vi "Historical Data Access Server.vi"() -> ()   [LabVIEW 2019, in "OPC UA Demo.lvlib"]
doc: "Demonstrates the use of the <B>OPC UA Historical Data Access</B> functionality as an OPC UA server."
uses:
  OPC UA Demo.lvlib
  <vilib>/OPCUA/controls/Data Type.ctl
  <vilib>/OPCUA/controls/Historical Access.ctl
  <vilib>/OPCUA/server/Write Double.vi
  <vilib>/OPCUA/NI OPC UA Server.lvlib
  <vilib>/ptbypt/NI_PtbyPt.lvlib
panel:
  out "Node0":dbl(graph)
  out "Node1":dbl(graph)
  in  "queue size":u32=2000
  in  "stop":bool
  out "Node2":dbl(graph)
  out "server endpoint URL":string
  # "Overview: Demonstrates the use of the OPC UA Historical Data Access functionality as an OPC UA server.\nRequirements: \n1. LabVIEW OPC UA Toolkit\n2. Run this VI on RT targets or Windows\nInstructions:\n1. Adjust queue size to change the buffer size of history data.\n2. Run the VI.\n3. Run Historical Data Access Client.vi in OPC UA Demo.lvproj."
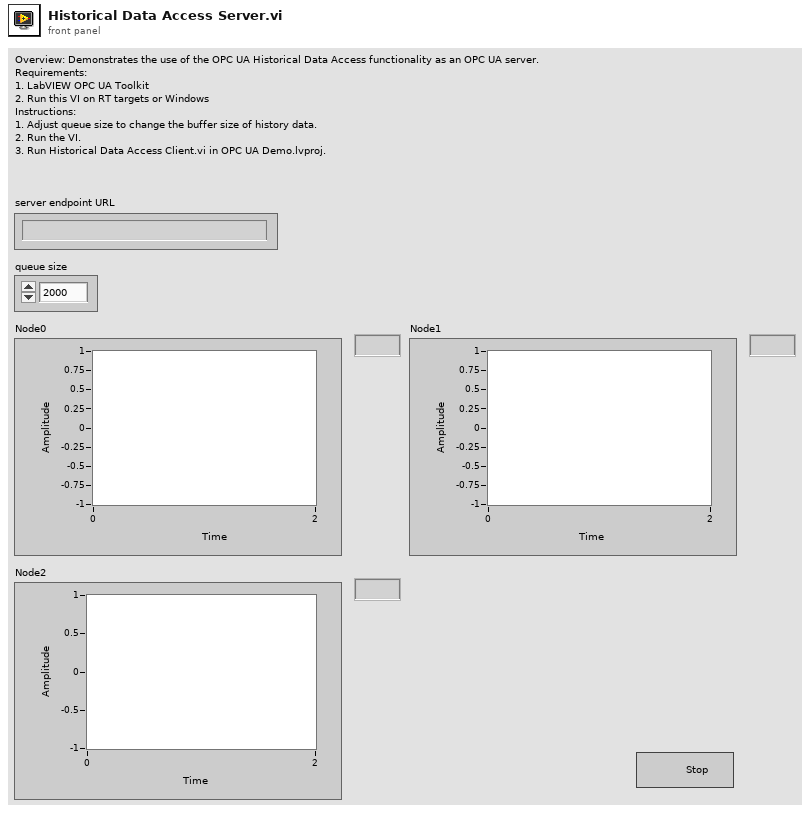
[diagram p1: front panel]
types:
  T1 = typedef "Historical Access.ctl" = cluster{"enable":bool, "queue size (1000)":u32}
  T2 = typedef "Data Type.ctl" = u16
  T3 = cluster{"name":string, "data type":T2, "access level":u16, "description":string}
  T4 = typedef "OPC UA Server Refnum.ctl" = refnum<k21>
  T5 = typedef "NodeId.ctl" = string
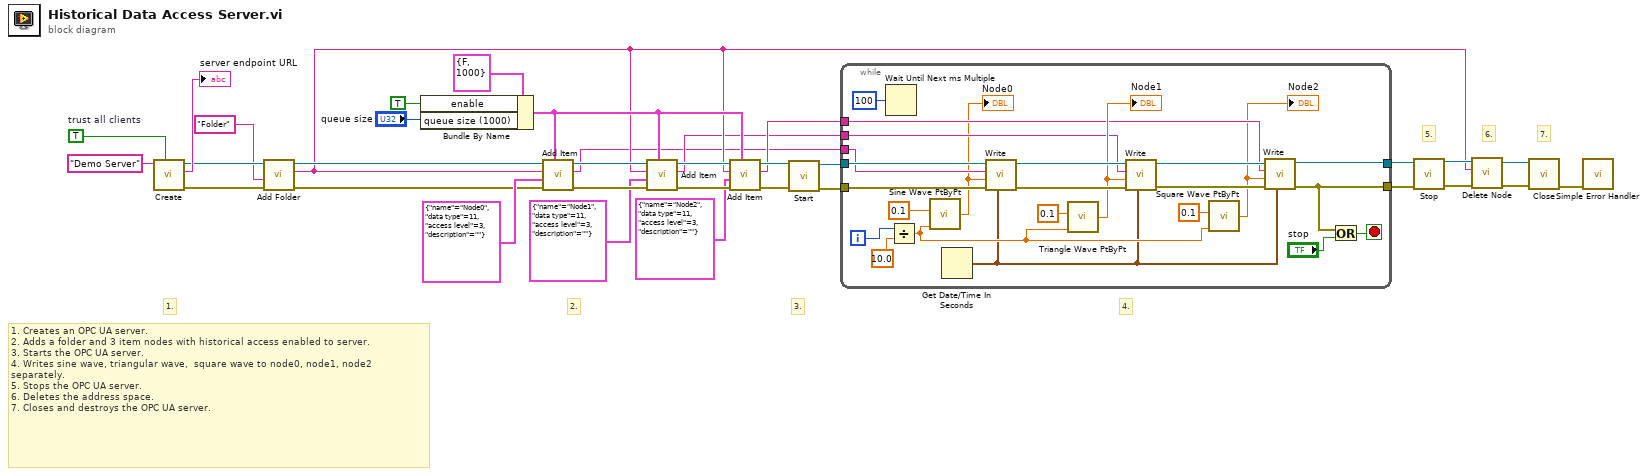
[diagram p0: block diagram]
diagram:
  w1 = TRUE  # trust all clients
  # "7."
  # "6."
  # "5."
  # "4."
  # "3."
  # "2."
  # "1."
  # "1. Creates an OPC UA server.\n2. Adds a folder and 3 item nodes with historical access enabled to server.\n3. Starts the OPC UA server.\n4. Writes sine wave, triangular wave,  square wave to node0, node1, node2 separately. \n5. Stops the OPC UA server.\n6. Deletes the address space.\n7. Closes and destroys the OPC UA server."
  n1 = call <vilib>:"Create.vi"("trust all clients (F)"=w1, "OPC UA server name"="Demo Server") -> ("error out"=w31:errorcluster, "server endpoint URL"=→"server endpoint URL":string, "OPC UA server refnum out"=w32:T4)  [unwired: 7 in]
  n2 = call <vilib>:"Add Folder.vi"("error in (no error)"=w31, "folder name"="Folder", "OPC UA server refnum in"=w32) -> ("error out"=w27:errorcluster, "folder node ID"=w6:T5, "OPC UA server refnum out"=w28:T4)  [unwired: 5 in]
  n3 = Bundle By Name(cluster=T1 {"enable"=FALSE, "queue size (1000)"=1000} ("historical access"), "enable"=TRUE, "queue size (1000)"="queue size") -> (w11:T1)
  n4 = call <vilib>:"Add Item.vi"("historical access"=w11, "error in (no error)"=w27, "item"=T3 {"name"="Node0", "data type"=11, "access level"=3, "description"=""}, "parent folder node ID"=w6, "OPC UA server refnum in"=w28) -> ("error out"=w15:errorcluster, "item node ID"=w2:T5, "OPC UA server refnum out"=w14:T4)  [unwired: 2 in, 1 out]
  n5 = call <vilib>:"Add Item.vi"("historical access"=w11, "error in (no error)"=w15, "item"=T3 {"name"="Node1", "data type"=11, "access level"=3, "description"=""}, "parent folder node ID"=w6, "OPC UA server refnum in"=w14) -> ("error out"=w8:errorcluster, "item node ID"=w3:T5, "OPC UA server refnum out"=w12:T4)  [unwired: 2 in, 1 out]
  n6 = call <vilib>:"Add Item.vi"("historical access"=w11, "error in (no error)"=w8, "item"=T3 {"name"="Node2", "data type"=11, "access level"=3, "description"=""}, "parent folder node ID"=w6, "OPC UA server refnum in"=w12) -> ("error out"=w9:errorcluster, "item node ID"=w4:T5, "OPC UA server refnum out"=w10:T4)  [unwired: 2 in, 1 out]
  n7 = call <vilib>:"Start.vi"("error in (no error)"=w9, "OPC UA server refnum in"=w10) -> ("error out"=w23:errorcluster, "OPC UA server refnum out"=w24:T4)  [unwired: 7 in, 1 out]
  n8 = while {
    tunnel: w24 -> [w58]
    tunnel: w23 -> [w56]
    tunnel: [w38] -> w25
    tunnel: [w48] -> w26
    tunnel: w4 -> [w41]
    tunnel: w3 -> [w42]
    tunnel: w2 -> [w43]
    i -> [w55]
    stop <- w39 stop-if-true
    n9 = Wait Until Next ms Multiple(millisecond multiple=u32 100) -> ()  [unwired: 1 out]
    n10 = Divide(x=w55, y=10.0 ("frequency")) -> (x/y=w46:dbl)
    n11 = call <vilib>:"Sine Wave PtByPt.vi"("time"=w46, "frequency"=0.1) -> ("sine wave"=w36:dbl)  [unwired: 2 in]
    "Node0" <- w36
    n12 = Get Date/Time In Seconds() -> (seconds since 1Jan1904=w37:timestamp)
    n13 = call-poly <vilib>:"Write.vi"("timestamp (current time)"=w37, "error in (no error)"=w56, "value"=w36, "node ID"=w43, "OPC UA server refnum in"=w58) -> ("error out"=w51:errorcluster, "OPC UA server refnum out"=w52:T4)  [unwired: 4 in, 1 out]
    n14 = call <vilib>:"Triangle Wave PtByPt.vi"("time"=w46, "frequency"=0.1) -> ("triangle wave"=w44:dbl)  [unwired: 2 in]
    "Node1" <- w44
    n15 = call-poly <vilib>:"Write.vi"("timestamp (current time)"=w37, "error in (no error)"=w51, "value"=w44, "node ID"=w42, "OPC UA server refnum in"=w52) -> ("error out"=w50:errorcluster, "OPC UA server refnum out"=w49:T4)  [unwired: 4 in, 1 out]
    n16 = call <vilib>:"Square Wave PtByPt.vi"("frequency"=0.1, "time"=w46) -> ("square wave"=w35:dbl)  [unwired: 3 in]
    "Node2" <- w35
    n17 = call-poly <vilib>:"Write.vi"("timestamp (current time)"=w37, "error in (no error)"=w50, "value"=w35, "node ID"=w41, "OPC UA server refnum in"=w49) -> ("error out"=w38:errorcluster, "OPC UA server refnum out"=w48:T4)  [unwired: 4 in, 1 out]
    n18 = Or(x=w38, y="stop") -> (x .or. y?=w39:bool)
  }
  n19 = call <vilib>:"Stop.vi"("error in (no error)"=w25, "OPC UA server refnum in"=w26) -> ("error out"=w21:errorcluster, "OPC UA server refnum out"=w18:T4)  [unwired: 8 in]
  n20 = call <vilib>:"Delete Node.vi"("error in (no error)"=w21, "node ID"=w6, "OPC UA server refnum in"=w18) -> ("error out"=w20:errorcluster, "OPC UA server refnum out"=w19:T4)  [unwired: 7 in]
  n21 = call <vilib>:"Close.vi"("error in (no error)"=w20, "OPC UA server refnum in"=w19) -> ("error out"=w22:errorcluster)  [unwired: 9 in]
  n22 = call <vilib>:"Simple Error Handler.vi"("error in (no error)"=w22) -> ()  [unwired: 4 in, 5 out]
